vi "Global 1.vi"() -> ()   [LabVIEW 2019]
panel:
  out "Numeric":dbl
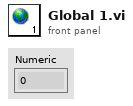
[diagram p1: front panel]
diagram:
